vi "Read Trace.vi"(0 "VISA resource name":refnum<visa-resource-name>, 1 "Data Source (0: Data Trace)":u16(ring) items=["Data Trace", "Memory Trace"], 2 "Data Type (0: Formatted)":T1(ring), 5 "Measurement Type (6: Phase Noise)":u16(ring)=6 items=["AM Noise"=1, "Baseband Noise"=2, "Freq/Power"=3, "Spectrum"=4, "Transient"=5, "Phase Noise"=6, "User"=7], 7 "Select Trace (1: 1)":u16(ring)=1 items=["1"=1, "2"=2, "3"=3, "4"=4, "5"=5, "6"=6, "7"=7, "8"=8], 11 "error in (no error)":errorcluster, 12 "Maximum Time (10000 ms)":u32=10000) -> (4 "VISA resource name out":refnum<visa-resource-name>, 6 "Measurements":dbl[](array[numeric]) format="%^#_9g", 15 "error out":errorcluster)   [LabVIEW 2011, in "Agilent E5052X.lvlib"]
doc: "Reads formatted trace data from the instrument. \n\n<b>Note: </b>\n\nIt can read either data from current trace or from trace stored in memory."
uses:
  Agilent E5052X.lvlib
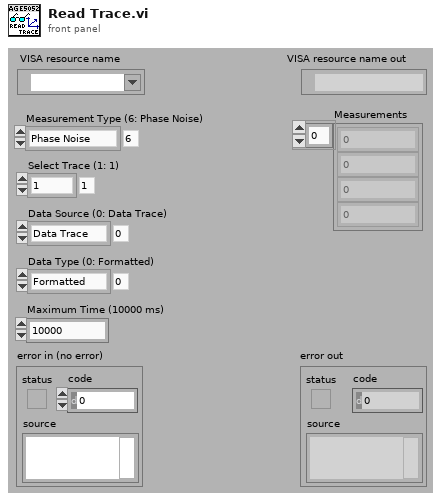
[diagram p1: front panel]
types:
  T1 = enum16{"Formatted", "Unformatted", "Power", "Spurious"}
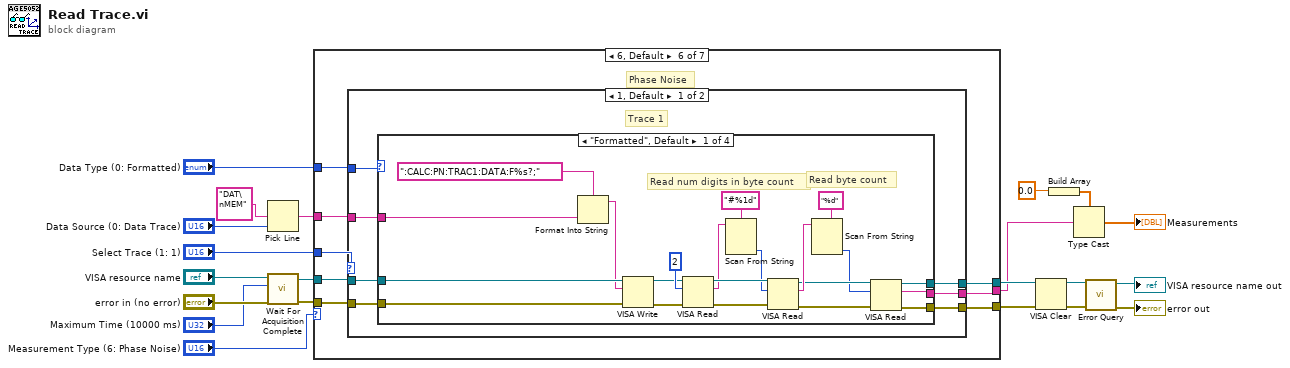
[diagram p0: block diagram]
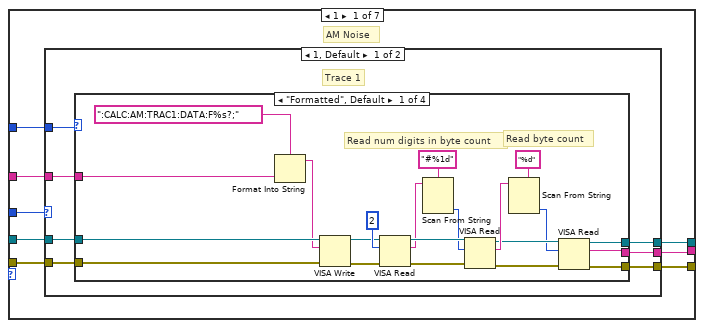
[diagram p2: hidden frame]
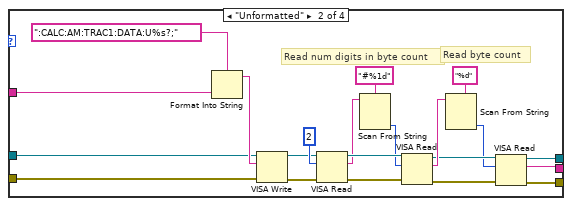
[diagram p3: hidden frame]
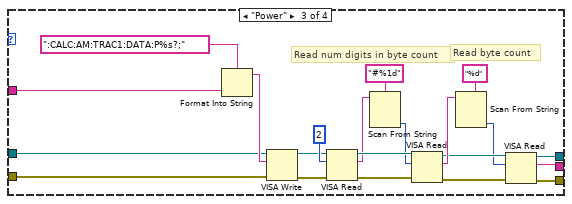
[diagram p4: hidden frame]
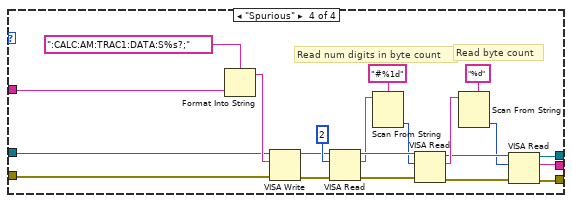
[diagram p5: hidden frame]
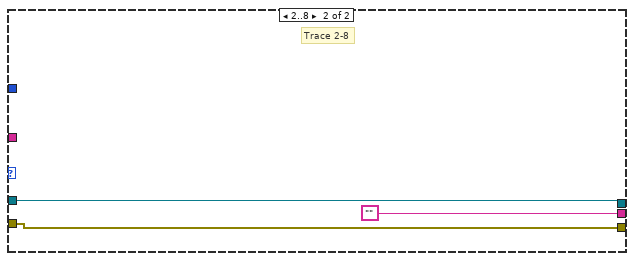
[diagram p6: hidden frame]
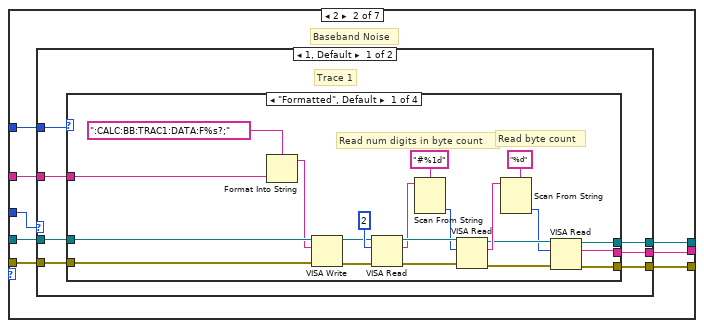
[diagram p7: hidden frame]
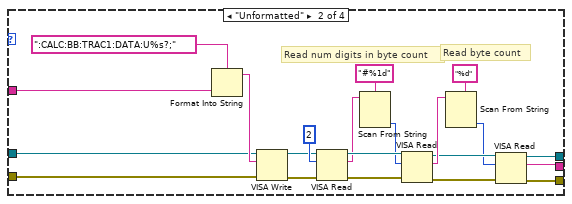
[diagram p8: hidden frame]
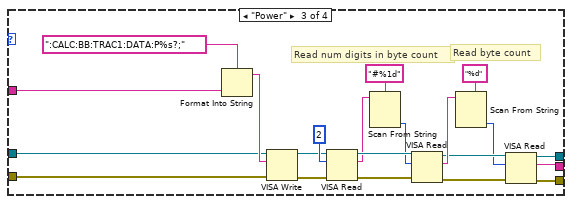
[diagram p9: hidden frame]
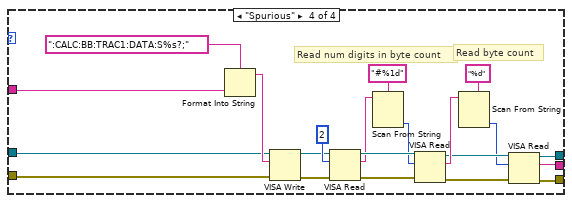
[diagram p10: hidden frame]
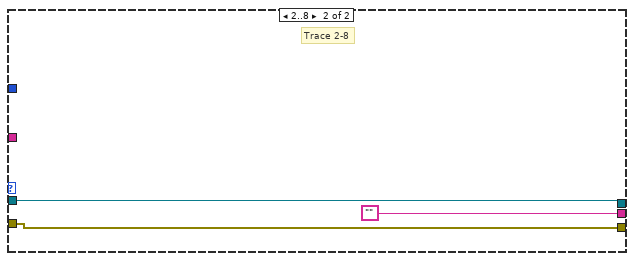
[diagram p11: hidden frame]
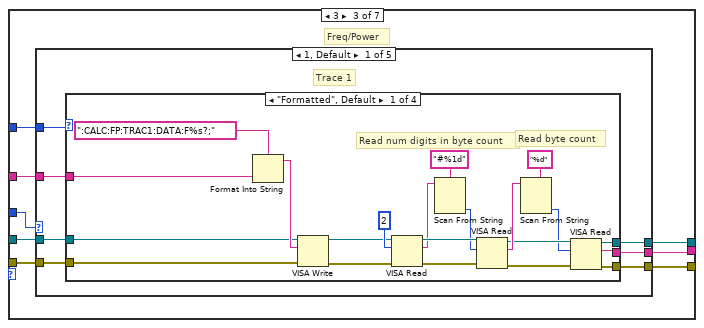
[diagram p12: hidden frame]
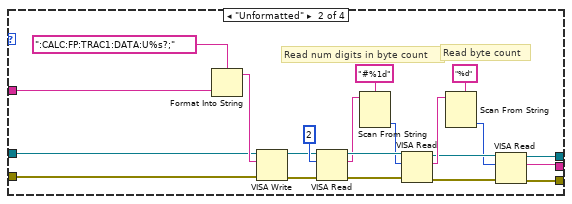
[diagram p13: hidden frame]
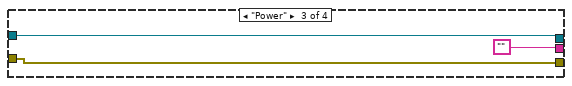
[diagram p14: hidden frame]
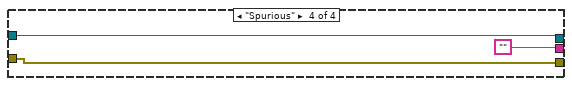
[diagram p15: hidden frame]
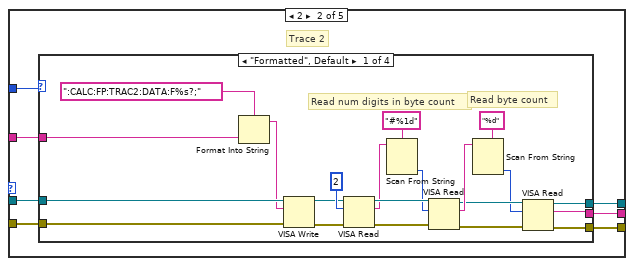
[diagram p16: hidden frame]
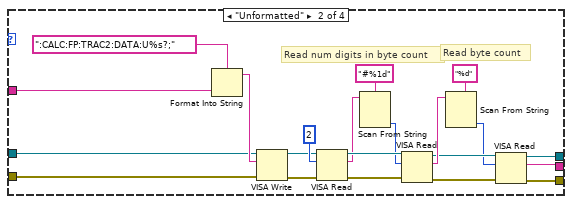
[diagram p17: hidden frame]
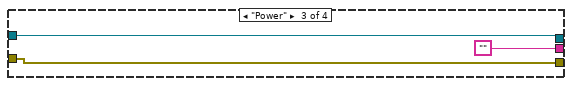
[diagram p18: hidden frame]
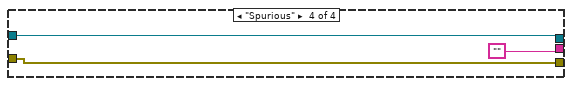
[diagram p19: hidden frame]
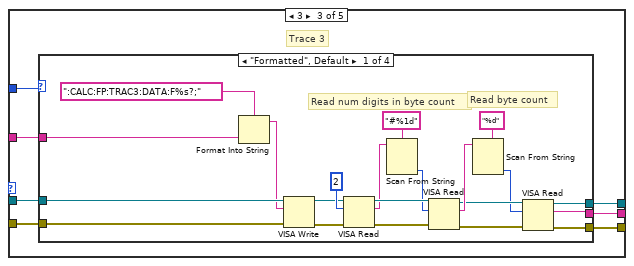
[diagram p20: hidden frame]
diagram:
  n1 = Pick Line(multi-line string="DAT\nMEM", line index="Data Source (0: Data Trace)") -> (output string=w14:string)  [unwired: 1 in]
  n2 = call "Wait For Acquisition Complete.vi"("error in (no error)"="error in (no error)", "Maximum Time (10000)"="Maximum Time (10000 ms)", "VISA resource name"="VISA resource name") -> ("error out"=w8:errorcluster, "VISA resource name out"=w9:refnum<visa-resource-name>)  [unwired: 7 in]
  n3 = case shown="6, Default" "Measurement Type (6: Phase Noise)" {
    tunnel: "Select Trace (1: 1)" -> [w29 w129 w231 w462 w528 w759 w861]
    tunnel: w14 -> [w28 w130 w232 w463 w529 w760 w862]
    tunnel: "Data Type (0: Formatted)" -> [w27 w131 w233 w464 w530 w761 w863]
    tunnel: w9 -> [w26 w128 w230 w461 w527 w758 w860]
    tunnel: w8 -> [w25 w127 w229 w460 w526 w757 w859]
    tunnel: [w24 w126 w228 w459 w525 w756 w858] -> w13
    tunnel: [w23 w124 w226 w457 w523 w754 w856] -> w12
    tunnel: [w22 w125 w227 w458 w524 w755 w857] -> w2
    frame 1 {
      # "AM Noise"
      n4 = case shown="1, Default" w29 {
        tunnel: w28 -> [w35 _]
        tunnel: w27 -> [w36 _]
        tunnel: w26 -> [w34 w122]
        tunnel: w25 -> [w33 w121]
        tunnel: [w32 w122] -> w24
        tunnel: [w31 w121] -> w23
        tunnel: [w30 ""] -> w22
        frame 1, Default {
          # "Trace 1"
          n5 = case shown="\"Formatted\", Default" w36 {
            tunnel: w35 -> [w56 w63 w84 w105]
            tunnel: w34 -> [w55 w62 w83 w104]
            tunnel: w33 -> [w54 w61 w82 w103]
            tunnel: [w52 w60 w81 w102] -> w32
            tunnel: [w51 w59 w79 w101] -> w31
            tunnel: [w50 w58 w80 w100] -> w30
            frame "Formatted", Default {
              # "Read num digits in byte count"
              # "Read byte count"
              n6 = Format Into String(format string=":CALC:AM:TRAC1:DATA:F%s?;", w56) -> (resulting string=w53:string)  [unwired: 2 in, 1 out]
              n7 = VISA Write(VISA resource name=w55, write buffer=w53, error in (no error)=w54) -> (VISA resource name out=w41:refnum<visa-resource-name>, error out=w40:errorcluster)  [unwired: 1 out]
              n8 = VISA Read(VISA resource name=w41, byte count=u32 2, error in (no error)=w40) -> (VISA resource name out=w46:refnum<visa-resource-name>, read buffer=w42:string, error out=w47:errorcluster)  [unwired: 1 out]
              n9 = Scan From String(format string="#%1d", input string=w42) -> (output 1=w45:i32)  [unwired: 3 in, 3 out]
              n10 = VISA Read(VISA resource name=w46, byte count=w45, error in (no error)=w47) -> (VISA resource name out=w39:refnum<visa-resource-name>, read buffer=w44:string, error out=w38:errorcluster)  [unwired: 1 out]
              n11 = Scan From String(format string="%d", input string=w44) -> (output 1=w37:i32)  [unwired: 3 in, 3 out]
              n12 = VISA Read(VISA resource name=w39, byte count=w37, error in (no error)=w38) -> (VISA resource name out=w52:refnum<visa-resource-name>, read buffer=w50:string, error out=w51:errorcluster)  [unwired: 1 out]
            }
            frame "Unformatted" {
              # "Read num digits in byte count"
              # "Read byte count"
              n13 = Format Into String(format string=":CALC:AM:TRAC1:DATA:U%s?;", w63) -> (resulting string=w77:string)  [unwired: 2 in, 1 out]
              n14 = VISA Write(VISA resource name=w62, write buffer=w77, error in (no error)=w61) -> (VISA resource name out=w68:refnum<visa-resource-name>, error out=w67:errorcluster)  [unwired: 1 out]
              n15 = VISA Read(VISA resource name=w68, byte count=u32 2, error in (no error)=w67) -> (VISA resource name out=w73:refnum<visa-resource-name>, read buffer=w69:string, error out=w74:errorcluster)  [unwired: 1 out]
              n16 = Scan From String(format string="#%1d", input string=w69) -> (output 1=w72:i32)  [unwired: 3 in, 3 out]
              n17 = VISA Read(VISA resource name=w73, byte count=w72, error in (no error)=w74) -> (VISA resource name out=w66:refnum<visa-resource-name>, read buffer=w71:string, error out=w65:errorcluster)  [unwired: 1 out]
              n18 = Scan From String(format string="%d", input string=w71) -> (output 1=w64:i32)  [unwired: 3 in, 3 out]
              n19 = VISA Read(VISA resource name=w66, byte count=w64, error in (no error)=w65) -> (VISA resource name out=w60:refnum<visa-resource-name>, read buffer=w58:string, error out=w59:errorcluster)  [unwired: 1 out]
            }
            frame "Power" {
              # "Read num digits in byte count"
              # "Read byte count"
              n20 = Format Into String(format string=":CALC:AM:TRAC1:DATA:P%s?;", w84) -> (resulting string=w98:string)  [unwired: 2 in, 1 out]
              n21 = VISA Write(VISA resource name=w83, write buffer=w98, error in (no error)=w82) -> (VISA resource name out=w89:refnum<visa-resource-name>, error out=w88:errorcluster)  [unwired: 1 out]
              n22 = VISA Read(VISA resource name=w89, byte count=u32 2, error in (no error)=w88) -> (VISA resource name out=w94:refnum<visa-resource-name>, read buffer=w90:string, error out=w95:errorcluster)  [unwired: 1 out]
              n23 = Scan From String(format string="#%1d", input string=w90) -> (output 1=w93:i32)  [unwired: 3 in, 3 out]
              n24 = VISA Read(VISA resource name=w94, byte count=w93, error in (no error)=w95) -> (VISA resource name out=w87:refnum<visa-resource-name>, read buffer=w92:string, error out=w86:errorcluster)  [unwired: 1 out]
              n25 = Scan From String(format string="%d", input string=w92) -> (output 1=w85:i32)  [unwired: 3 in, 3 out]
              n26 = VISA Read(VISA resource name=w87, byte count=w85, error in (no error)=w86) -> (VISA resource name out=w81:refnum<visa-resource-name>, read buffer=w80:string, error out=w79:errorcluster)  [unwired: 1 out]
            }
            frame "Spurious" {
              # "Read num digits in byte count"
              # "Read byte count"
              n27 = Format Into String(format string=":CALC:AM:TRAC1:DATA:S%s?;", w105) -> (resulting string=w119:string)  [unwired: 2 in, 1 out]
              n28 = VISA Write(VISA resource name=w104, write buffer=w119, error in (no error)=w103) -> (VISA resource name out=w110:refnum<visa-resource-name>, error out=w109:errorcluster)  [unwired: 1 out]
              n29 = VISA Read(VISA resource name=w110, byte count=u32 2, error in (no error)=w109) -> (VISA resource name out=w115:refnum<visa-resource-name>, read buffer=w111:string, error out=w116:errorcluster)  [unwired: 1 out]
              n30 = Scan From String(format string="#%1d", input string=w111) -> (output 1=w114:i32)  [unwired: 3 in, 3 out]
              n31 = VISA Read(VISA resource name=w115, byte count=w114, error in (no error)=w116) -> (VISA resource name out=w108:refnum<visa-resource-name>, read buffer=w113:string, error out=w107:errorcluster)  [unwired: 1 out]
              n32 = Scan From String(format string="%d", input string=w113) -> (output 1=w106:i32)  [unwired: 3 in, 3 out]
              n33 = VISA Read(VISA resource name=w108, byte count=w106, error in (no error)=w107) -> (VISA resource name out=w102:refnum<visa-resource-name>, read buffer=w100:string, error out=w101:errorcluster)  [unwired: 1 out]
            }
          }
        }
        frame 2..8 {
          # "Trace 2-8"
        }
      }
    }
    frame 2 {
      # "Baseband Noise"
      n34 = case shown="1, Default" w129 {
        tunnel: w130 -> [w137 _]
        tunnel: w131 -> [w138 _]
        tunnel: w128 -> [w136 w224]
        tunnel: w127 -> [w135 w223]
        tunnel: [w134 w224] -> w126
        tunnel: [w133 w223] -> w124
        tunnel: [w132 ""] -> w125
        frame 1, Default {
          # "Trace 1"
          n35 = case shown="\"Formatted\", Default" w138 {
            tunnel: w137 -> [w158 w165 w186 w207]
            tunnel: w136 -> [w157 w164 w185 w206]
            tunnel: w135 -> [w156 w163 w184 w205]
            tunnel: [w154 w162 w183 w204] -> w134
            tunnel: [w153 w161 w181 w203] -> w133
            tunnel: [w152 w160 w182 w202] -> w132
            frame "Formatted", Default {
              # "Read num digits in byte count"
              # "Read byte count"
              n36 = Format Into String(format string=":CALC:BB:TRAC1:DATA:F%s?;", w158) -> (resulting string=w155:string)  [unwired: 2 in, 1 out]
              n37 = VISA Write(VISA resource name=w157, write buffer=w155, error in (no error)=w156) -> (VISA resource name out=w143:refnum<visa-resource-name>, error out=w142:errorcluster)  [unwired: 1 out]
              n38 = VISA Read(VISA resource name=w143, byte count=u32 2, error in (no error)=w142) -> (VISA resource name out=w148:refnum<visa-resource-name>, read buffer=w144:string, error out=w149:errorcluster)  [unwired: 1 out]
              n39 = Scan From String(format string="#%1d", input string=w144) -> (output 1=w147:i32)  [unwired: 3 in, 3 out]
              n40 = VISA Read(VISA resource name=w148, byte count=w147, error in (no error)=w149) -> (VISA resource name out=w141:refnum<visa-resource-name>, read buffer=w146:string, error out=w140:errorcluster)  [unwired: 1 out]
              n41 = Scan From String(format string="%d", input string=w146) -> (output 1=w139:i32)  [unwired: 3 in, 3 out]
              n42 = VISA Read(VISA resource name=w141, byte count=w139, error in (no error)=w140) -> (VISA resource name out=w154:refnum<visa-resource-name>, read buffer=w152:string, error out=w153:errorcluster)  [unwired: 1 out]
            }
            frame "Unformatted" {
              # "Read num digits in byte count"
              # "Read byte count"
              n43 = Format Into String(format string=":CALC:BB:TRAC1:DATA:U%s?;", w165) -> (resulting string=w179:string)  [unwired: 2 in, 1 out]
              n44 = VISA Write(VISA resource name=w164, write buffer=w179, error in (no error)=w163) -> (VISA resource name out=w170:refnum<visa-resource-name>, error out=w169:errorcluster)  [unwired: 1 out]
              n45 = VISA Read(VISA resource name=w170, byte count=u32 2, error in (no error)=w169) -> (VISA resource name out=w175:refnum<visa-resource-name>, read buffer=w171:string, error out=w176:errorcluster)  [unwired: 1 out]
              n46 = Scan From String(format string="#%1d", input string=w171) -> (output 1=w174:i32)  [unwired: 3 in, 3 out]
              n47 = VISA Read(VISA resource name=w175, byte count=w174, error in (no error)=w176) -> (VISA resource name out=w168:refnum<visa-resource-name>, read buffer=w173:string, error out=w167:errorcluster)  [unwired: 1 out]
              n48 = Scan From String(format string="%d", input string=w173) -> (output 1=w166:i32)  [unwired: 3 in, 3 out]
              n49 = VISA Read(VISA resource name=w168, byte count=w166, error in (no error)=w167) -> (VISA resource name out=w162:refnum<visa-resource-name>, read buffer=w160:string, error out=w161:errorcluster)  [unwired: 1 out]
            }
            frame "Power" {
              # "Read num digits in byte count"
              # "Read byte count"
              n50 = Format Into String(format string=":CALC:BB:TRAC1:DATA:P%s?;", w186) -> (resulting string=w200:string)  [unwired: 2 in, 1 out]
              n51 = VISA Write(VISA resource name=w185, write buffer=w200, error in (no error)=w184) -> (VISA resource name out=w191:refnum<visa-resource-name>, error out=w190:errorcluster)  [unwired: 1 out]
              n52 = VISA Read(VISA resource name=w191, byte count=u32 2, error in (no error)=w190) -> (VISA resource name out=w196:refnum<visa-resource-name>, read buffer=w192:string, error out=w197:errorcluster)  [unwired: 1 out]
              n53 = Scan From String(format string="#%1d", input string=w192) -> (output 1=w195:i32)  [unwired: 3 in, 3 out]
              n54 = VISA Read(VISA resource name=w196, byte count=w195, error in (no error)=w197) -> (VISA resource name out=w189:refnum<visa-resource-name>, read buffer=w194:string, error out=w188:errorcluster)  [unwired: 1 out]
              n55 = Scan From String(format string="%d", input string=w194) -> (output 1=w187:i32)  [unwired: 3 in, 3 out]
              n56 = VISA Read(VISA resource name=w189, byte count=w187, error in (no error)=w188) -> (VISA resource name out=w183:refnum<visa-resource-name>, read buffer=w182:string, error out=w181:errorcluster)  [unwired: 1 out]
            }
            frame "Spurious" {
              # "Read num digits in byte count"
              # "Read byte count"
              n57 = Format Into String(format string=":CALC:BB:TRAC1:DATA:S%s?;", w207) -> (resulting string=w221:string)  [unwired: 2 in, 1 out]
              n58 = VISA Write(VISA resource name=w206, write buffer=w221, error in (no error)=w205) -> (VISA resource name out=w212:refnum<visa-resource-name>, error out=w211:errorcluster)  [unwired: 1 out]
              n59 = VISA Read(VISA resource name=w212, byte count=u32 2, error in (no error)=w211) -> (VISA resource name out=w217:refnum<visa-resource-name>, read buffer=w213:string, error out=w218:errorcluster)  [unwired: 1 out]
              n60 = Scan From String(format string="#%1d", input string=w213) -> (output 1=w216:i32)  [unwired: 3 in, 3 out]
              n61 = VISA Read(VISA resource name=w217, byte count=w216, error in (no error)=w218) -> (VISA resource name out=w210:refnum<visa-resource-name>, read buffer=w215:string, error out=w209:errorcluster)  [unwired: 1 out]
              n62 = Scan From String(format string="%d", input string=w215) -> (output 1=w208:i32)  [unwired: 3 in, 3 out]
              n63 = VISA Read(VISA resource name=w210, byte count=w208, error in (no error)=w209) -> (VISA resource name out=w204:refnum<visa-resource-name>, read buffer=w202:string, error out=w203:errorcluster)  [unwired: 1 out]
            }
          }
        }
        frame 2..8 {
          # "Trace 2-8"
        }
      }
    }
    frame 3 {
      # "Freq/Power"
      n64 = case shown="1, Default" w231 {
        tunnel: w232 -> [w239 w294 w349 w404 _]
        tunnel: w233 -> [w240 w295 w350 w405 _]
        tunnel: w230 -> [w238 w293 w348 w403 w456]
        tunnel: w229 -> [w237 w292 w347 w402 w455]
        tunnel: [w236 w291 w346 w401 w456] -> w228
        tunnel: [w235 w290 w345 w400 w455] -> w226
        tunnel: [w234 w289 w344 w399 ""] -> w227
        frame 1, Default {
          # "Trace 1"
          n65 = case shown="\"Formatted\", Default" w240 {
            tunnel: w239 -> [w260 w267 _ _]
            tunnel: w238 -> [w242 w266 w285 w288]
            tunnel: w237 -> [w241 w265 w284 w287]
            tunnel: [w258 w264 w285 w288] -> w236
            tunnel: [w257 w263 w284 w287] -> w235
            tunnel: [w256 w262 "" ""] -> w234
            frame "Formatted", Default {
              # "Read num digits in byte count"
              # "Read byte count"
              n66 = Format Into String(format string=":CALC:FP:TRAC1:DATA:F%s?;", w260) -> (resulting string=w259:string)  [unwired: 2 in, 1 out]
              n67 = VISA Write(VISA resource name=w242, write buffer=w259, error in (no error)=w241) -> (VISA resource name out=w244:refnum<visa-resource-name>, error out=w243:errorcluster)  [unwired: 1 out]
              n68 = VISA Read(VISA resource name=w244, byte count=u32 2, error in (no error)=w243) -> (VISA resource name out=w252:refnum<visa-resource-name>, read buffer=w248:string, error out=w253:errorcluster)  [unwired: 1 out]
              n69 = Scan From String(format string="#%1d", input string=w248) -> (output 1=w251:i32)  [unwired: 3 in, 3 out]
              n70 = VISA Read(VISA resource name=w252, byte count=w251, error in (no error)=w253) -> (VISA resource name out=w247:refnum<visa-resource-name>, read buffer=w250:string, error out=w246:errorcluster)  [unwired: 1 out]
              n71 = Scan From String(format string="%d", input string=w250) -> (output 1=w245:i32)  [unwired: 3 in, 3 out]
              n72 = VISA Read(VISA resource name=w247, byte count=w245, error in (no error)=w246) -> (VISA resource name out=w258:refnum<visa-resource-name>, read buffer=w256:string, error out=w257:errorcluster)  [unwired: 1 out]
            }
            frame "Unformatted" {
              # "Read num digits in byte count"
              # "Read byte count"
              n73 = Format Into String(format string=":CALC:FP:TRAC1:DATA:U%s?;", w267) -> (resulting string=w281:string)  [unwired: 2 in, 1 out]
              n74 = VISA Write(VISA resource name=w266, write buffer=w281, error in (no error)=w265) -> (VISA resource name out=w272:refnum<visa-resource-name>, error out=w271:errorcluster)  [unwired: 1 out]
              n75 = VISA Read(VISA resource name=w272, byte count=u32 2, error in (no error)=w271) -> (VISA resource name out=w277:refnum<visa-resource-name>, read buffer=w273:string, error out=w278:errorcluster)  [unwired: 1 out]
              n76 = Scan From String(format string="#%1d", input string=w273) -> (output 1=w276:i32)  [unwired: 3 in, 3 out]
              n77 = VISA Read(VISA resource name=w277, byte count=w276, error in (no error)=w278) -> (VISA resource name out=w270:refnum<visa-resource-name>, read buffer=w275:string, error out=w269:errorcluster)  [unwired: 1 out]
              n78 = Scan From String(format string="%d", input string=w275) -> (output 1=w268:i32)  [unwired: 3 in, 3 out]
              n79 = VISA Read(VISA resource name=w270, byte count=w268, error in (no error)=w269) -> (VISA resource name out=w264:refnum<visa-resource-name>, read buffer=w262:string, error out=w263:errorcluster)  [unwired: 1 out]
            }
            frame "Power" {
            }
            frame "Spurious" {
            }
          }
        }
        frame 2 {
          # "Trace 2"
          n80 = case shown="\"Formatted\", Default" w295 {
            tunnel: w294 -> [w315 w322 _ _]
            tunnel: w293 -> [w314 w321 w340 w343]
            tunnel: w292 -> [w313 w320 w339 w342]
            tunnel: [w311 w319 w340 w343] -> w291
            tunnel: [w310 w318 w339 w342] -> w290
            tunnel: [w309 w317 "" ""] -> w289
            frame "Formatted", Default {
              # "Read num digits in byte count"
              # "Read byte count"
              n81 = Format Into String(format string=":CALC:FP:TRAC2:DATA:F%s?;", w315) -> (resulting string=w312:string)  [unwired: 2 in, 1 out]
              n82 = VISA Write(VISA resource name=w314, write buffer=w312, error in (no error)=w313) -> (VISA resource name out=w300:refnum<visa-resource-name>, error out=w299:errorcluster)  [unwired: 1 out]
              n83 = VISA Read(VISA resource name=w300, byte count=u32 2, error in (no error)=w299) -> (VISA resource name out=w305:refnum<visa-resource-name>, read buffer=w301:string, error out=w306:errorcluster)  [unwired: 1 out]
              n84 = Scan From String(format string="#%1d", input string=w301) -> (output 1=w304:i32)  [unwired: 3 in, 3 out]
              n85 = VISA Read(VISA resource name=w305, byte count=w304, error in (no error)=w306) -> (VISA resource name out=w298:refnum<visa-resource-name>, read buffer=w303:string, error out=w297:errorcluster)  [unwired: 1 out]
              n86 = Scan From String(format string="%d", input string=w303) -> (output 1=w296:i32)  [unwired: 3 in, 3 out]
              n87 = VISA Read(VISA resource name=w298, byte count=w296, error in (no error)=w297) -> (VISA resource name out=w311:refnum<visa-resource-name>, read buffer=w309:string, error out=w310:errorcluster)  [unwired: 1 out]
            }
            frame "Unformatted" {
              # "Read num digits in byte count"
              # "Read byte count"
              n88 = Format Into String(format string=":CALC:FP:TRAC2:DATA:U%s?;", w322) -> (resulting string=w336:string)  [unwired: 2 in, 1 out]
              n89 = VISA Write(VISA resource name=w321, write buffer=w336, error in (no error)=w320) -> (VISA resource name out=w327:refnum<visa-resource-name>, error out=w326:errorcluster)  [unwired: 1 out]
              n90 = VISA Read(VISA resource name=w327, byte count=u32 2, error in (no error)=w326) -> (VISA resource name out=w332:refnum<visa-resource-name>, read buffer=w328:string, error out=w333:errorcluster)  [unwired: 1 out]
              n91 = Scan From String(format string="#%1d", input string=w328) -> (output 1=w331:i32)  [unwired: 3 in, 3 out]
              n92 = VISA Read(VISA resource name=w332, byte count=w331, error in (no error)=w333) -> (VISA resource name out=w325:refnum<visa-resource-name>, read buffer=w330:string, error out=w324:errorcluster)  [unwired: 1 out]
              n93 = Scan From String(format string="%d", input string=w330) -> (output 1=w323:i32)  [unwired: 3 in, 3 out]
              n94 = VISA Read(VISA resource name=w325, byte count=w323, error in (no error)=w324) -> (VISA resource name out=w319:refnum<visa-resource-name>, read buffer=w317:string, error out=w318:errorcluster)  [unwired: 1 out]
            }
            frame "Power" {
            }
            frame "Spurious" {
            }
          }
        }
        frame 3 {
          # "Trace 3"
          n95 = case shown="\"Formatted\", Default" w350 {
            tunnel: w349 -> [w370 w377 _ _]
            tunnel: w348 -> [w369 w376 w395 w398]
            tunnel: w347 -> [w368 w375 w394 w397]
            tunnel: [w366 w374 w395 w398] -> w346
            tunnel: [w365 w373 w394 w397] -> w345
            tunnel: [w364 w372 "" ""] -> w344
            frame "Formatted", Default {
              # "Read num digits in byte count"
              # "Read byte count"
              n96 = Format Into String(format string=":CALC:FP:TRAC3:DATA:F%s?;", w370) -> (resulting string=w367:string)  [unwired: 2 in, 1 out]
              n97 = VISA Write(VISA resource name=w369, write buffer=w367, error in (no error)=w368) -> (VISA resource name out=w355:refnum<visa-resource-name>, error out=w354:errorcluster)  [unwired: 1 out]
              n98 = VISA Read(VISA resource name=w355, byte count=u32 2, error in (no error)=w354) -> (VISA resource name out=w360:refnum<visa-resource-name>, read buffer=w356:string, error out=w361:errorcluster)  [unwired: 1 out]
              n99 = Scan From String(format string="#%1d", input string=w356) -> (output 1=w359:i32)  [unwired: 3 in, 3 out]
              n100 = VISA Read(VISA resource name=w360, byte count=w359, error in (no error)=w361) -> (VISA resource name out=w353:refnum<visa-resource-name>, read buffer=w358:string, error out=w352:errorcluster)  [unwired: 1 out]
              n101 = Scan From String(format string="%d", input string=w358) -> (output 1=w351:i32)  [unwired: 3 in, 3 out]
              n102 = VISA Read(VISA resource name=w353, byte count=w351, error in (no error)=w352) -> (VISA resource name out=w366:refnum<visa-resource-name>, read buffer=w364:string, error out=w365:errorcluster)  [unwired: 1 out]
            }
            frame "Unformatted" {
              # "Read num digits in byte count"
              # "Read byte count"
              n103 = Format Into String(format string=":CALC:FP:TRAC3:DATA:U%s?;", w377) -> (resulting string=w391:string)  [unwired: 2 in, 1 out]
              n104 = VISA Write(VISA resource name=w376, write buffer=w391, error in (no error)=w375) -> (VISA resource name out=w382:refnum<visa-resource-name>, error out=w381:errorcluster)  [unwired: 1 out]
              n105 = VISA Read(VISA resource name=w382, byte count=u32 2, error in (no error)=w381) -> (VISA resource name out=w387:refnum<visa-resource-name>, read buffer=w383:string, error out=w388:errorcluster)  [unwired: 1 out]
              n106 = Scan From String(format string="#%1d", input string=w383) -> (output 1=w386:i32)  [unwired: 3 in, 3 out]
              n107 = VISA Read(VISA resource name=w387, byte count=w386, error in (no error)=w388) -> (VISA resource name out=w380:refnum<visa-resource-name>, read buffer=w385:string, error out=w379:errorcluster)  [unwired: 1 out]
              n108 = Scan From String(format string="%d", input string=w385) -> (output 1=w378:i32)  [unwired: 3 in, 3 out]
              n109 = VISA Read(VISA resource name=w380, byte count=w378, error in (no error)=w379) -> (VISA resource name out=w374:refnum<visa-resource-name>, read buffer=w372:string, error out=w373:errorcluster)  [unwired: 1 out]
            }
            frame "Power" {
            }
            frame "Spurious" {
            }
          }
        }
        frame 4 {
          # "Trace 4"
          n110 = case shown="\"Formatted\", Default" w405 {
            tunnel: w404 -> [w425 w432 _ _]
            tunnel: w403 -> [w424 w431 w450 w453]
            tunnel: w402 -> [w423 w430 w449 w452]
            tunnel: [w421 w429 w450 w453] -> w401
            tunnel: [w420 w428 w449 w452] -> w400
            tunnel: [w419 w427 "" ""] -> w399
            frame "Formatted", Default {
              # "Read num digits in byte count"
              # "Read byte count"
              n111 = Format Into String(format string=":CALC:FP:TRAC4:DATA:F%s?;", w425) -> (resulting string=w422:string)  [unwired: 2 in, 1 out]
              n112 = VISA Write(VISA resource name=w424, write buffer=w422, error in (no error)=w423) -> (VISA resource name out=w410:refnum<visa-resource-name>, error out=w409:errorcluster)  [unwired: 1 out]
              n113 = VISA Read(VISA resource name=w410, byte count=u32 2, error in (no error)=w409) -> (VISA resource name out=w415:refnum<visa-resource-name>, read buffer=w411:string, error out=w416:errorcluster)  [unwired: 1 out]
              n114 = Scan From String(format string="#%1d", input string=w411) -> (output 1=w414:i32)  [unwired: 3 in, 3 out]
              n115 = VISA Read(VISA resource name=w415, byte count=w414, error in (no error)=w416) -> (VISA resource name out=w408:refnum<visa-resource-name>, read buffer=w413:string, error out=w407:errorcluster)  [unwired: 1 out]
              n116 = Scan From String(format string="%d", input string=w413) -> (output 1=w406:i32)  [unwired: 3 in, 3 out]
              n117 = VISA Read(VISA resource name=w408, byte count=w406, error in (no error)=w407) -> (VISA resource name out=w421:refnum<visa-resource-name>, read buffer=w419:string, error out=w420:errorcluster)  [unwired: 1 out]
            }
            frame "Unformatted" {
              # "Read num digits in byte count"
              # "Read byte count"
              n118 = Format Into String(format string=":CALC:FP:TRAC4:DATA:U%s?;", w432) -> (resulting string=w446:string)  [unwired: 2 in, 1 out]
              n119 = VISA Write(VISA resource name=w431, write buffer=w446, error in (no error)=w430) -> (VISA resource name out=w437:refnum<visa-resource-name>, error out=w436:errorcluster)  [unwired: 1 out]
              n120 = VISA Read(VISA resource name=w437, byte count=u32 2, error in (no error)=w436) -> (VISA resource name out=w442:refnum<visa-resource-name>, read buffer=w438:string, error out=w443:errorcluster)  [unwired: 1 out]
              n121 = Scan From String(format string="#%1d", input string=w438) -> (output 1=w441:i32)  [unwired: 3 in, 3 out]
              n122 = VISA Read(VISA resource name=w442, byte count=w441, error in (no error)=w443) -> (VISA resource name out=w435:refnum<visa-resource-name>, read buffer=w440:string, error out=w434:errorcluster)  [unwired: 1 out]
              n123 = Scan From String(format string="%d", input string=w440) -> (output 1=w433:i32)  [unwired: 3 in, 3 out]
              n124 = VISA Read(VISA resource name=w435, byte count=w433, error in (no error)=w434) -> (VISA resource name out=w429:refnum<visa-resource-name>, read buffer=w427:string, error out=w428:errorcluster)  [unwired: 1 out]
            }
            frame "Power" {
            }
            frame "Spurious" {
            }
          }
        }
        frame 5..8 {
        }
      }
    }
    frame 4 {
      # "Spectrum"
      n125 = case shown="1, Default" w462 {
        tunnel: w463 -> [w470 _]
        tunnel: w464 -> [w471 _]
        tunnel: w461 -> [w469 w521]
        tunnel: w460 -> [w468 w520]
        tunnel: [w467 w521] -> w459
        tunnel: [w466 w520] -> w457
        tunnel: [w465 ""] -> w458
        frame 1, Default {
          # "Trace 1"
          n126 = case shown="\"Formatted\", Default" w471 {
            tunnel: w470 -> [w491 w498 _ _]
            tunnel: w469 -> [w490 w497 w516 w519]
            tunnel: w468 -> [w489 w496 w515 w518]
            tunnel: [w487 w495 w516 w519] -> w467
            tunnel: [w486 w494 w515 w518] -> w466
            tunnel: [w485 w493 "" ""] -> w465
            frame "Formatted", Default {
              # "Read num digits in byte count"
              # "Read byte count"
              n127 = Format Into String(format string=":CALC:SP:TRAC1:DATA:F%s?;", w491) -> (resulting string=w488:string)  [unwired: 2 in, 1 out]
              n128 = VISA Write(VISA resource name=w490, write buffer=w488, error in (no error)=w489) -> (VISA resource name out=w476:refnum<visa-resource-name>, error out=w475:errorcluster)  [unwired: 1 out]
              n129 = VISA Read(VISA resource name=w476, byte count=u32 2, error in (no error)=w475) -> (VISA resource name out=w481:refnum<visa-resource-name>, read buffer=w477:string, error out=w482:errorcluster)  [unwired: 1 out]
              n130 = Scan From String(format string="#%1d", input string=w477) -> (output 1=w480:i32)  [unwired: 3 in, 3 out]
              n131 = VISA Read(VISA resource name=w481, byte count=w480, error in (no error)=w482) -> (VISA resource name out=w474:refnum<visa-resource-name>, read buffer=w479:string, error out=w473:errorcluster)  [unwired: 1 out]
              n132 = Scan From String(format string="%d", input string=w479) -> (output 1=w472:i32)  [unwired: 3 in, 3 out]
              n133 = VISA Read(VISA resource name=w474, byte count=w472, error in (no error)=w473) -> (VISA resource name out=w487:refnum<visa-resource-name>, read buffer=w485:string, error out=w486:errorcluster)  [unwired: 1 out]
            }
            frame "Unformatted" {
              # "Read num digits in byte count"
              # "Read byte count"
              n134 = Format Into String(format string=":CALC:SP:TRAC1:DATA:U%s?;", w498) -> (resulting string=w512:string)  [unwired: 2 in, 1 out]
              n135 = VISA Write(VISA resource name=w497, write buffer=w512, error in (no error)=w496) -> (VISA resource name out=w503:refnum<visa-resource-name>, error out=w502:errorcluster)  [unwired: 1 out]
              n136 = VISA Read(VISA resource name=w503, byte count=u32 2, error in (no error)=w502) -> (VISA resource name out=w508:refnum<visa-resource-name>, read buffer=w504:string, error out=w509:errorcluster)  [unwired: 1 out]
              n137 = Scan From String(format string="#%1d", input string=w504) -> (output 1=w507:i32)  [unwired: 3 in, 3 out]
              n138 = VISA Read(VISA resource name=w508, byte count=w507, error in (no error)=w509) -> (VISA resource name out=w501:refnum<visa-resource-name>, read buffer=w506:string, error out=w500:errorcluster)  [unwired: 1 out]
              n139 = Scan From String(format string="%d", input string=w506) -> (output 1=w499:i32)  [unwired: 3 in, 3 out]
              n140 = VISA Read(VISA resource name=w501, byte count=w499, error in (no error)=w500) -> (VISA resource name out=w495:refnum<visa-resource-name>, read buffer=w493:string, error out=w494:errorcluster)  [unwired: 1 out]
            }
            frame "Power" {
            }
            frame "Spurious" {
            }
          }
        }
        frame 2..8 {
          # "Trace 2-8"
        }
      }
    }
    frame 5 {
      # "Transient"
      n141 = case shown="1, Default" w528 {
        tunnel: w529 -> [w536 w591 w646 w701 _]
        tunnel: w530 -> [w537 w592 w647 w702 _]
        tunnel: w527 -> [w535 w590 w645 w700 w753]
        tunnel: w526 -> [w534 w589 w644 w699 w752]
        tunnel: [w533 w588 w643 w698 w753] -> w525
        tunnel: [w532 w587 w642 w697 w752] -> w523
        tunnel: [w531 w586 w641 w696 ""] -> w524
        frame 1, Default {
          # "Trace 1"
          n142 = case shown="\"Formatted\", Default" w537 {
            tunnel: w536 -> [w557 w564 _ _]
            tunnel: w535 -> [w556 w563 w582 w585]
            tunnel: w534 -> [w555 w562 w581 w584]
            tunnel: [w553 w561 w582 w585] -> w533
            tunnel: [w552 w560 w581 w584] -> w532
            tunnel: [w551 w559 "" ""] -> w531
            frame "Formatted", Default {
              # "Read num digits in byte count"
              # "Read byte count"
              n143 = Format Into String(format string=":CALC:TR:TRAC1:DATA:F%s?;", w557) -> (resulting string=w554:string)  [unwired: 2 in, 1 out]
              n144 = VISA Write(VISA resource name=w556, write buffer=w554, error in (no error)=w555) -> (VISA resource name out=w542:refnum<visa-resource-name>, error out=w541:errorcluster)  [unwired: 1 out]
              n145 = VISA Read(VISA resource name=w542, byte count=u32 2, error in (no error)=w541) -> (VISA resource name out=w547:refnum<visa-resource-name>, read buffer=w543:string, error out=w548:errorcluster)  [unwired: 1 out]
              n146 = Scan From String(format string="#%1d", input string=w543) -> (output 1=w546:i32)  [unwired: 3 in, 3 out]
              n147 = VISA Read(VISA resource name=w547, byte count=w546, error in (no error)=w548) -> (VISA resource name out=w540:refnum<visa-resource-name>, read buffer=w545:string, error out=w539:errorcluster)  [unwired: 1 out]
              n148 = Scan From String(format string="%d", input string=w545) -> (output 1=w538:i32)  [unwired: 3 in, 3 out]
              n149 = VISA Read(VISA resource name=w540, byte count=w538, error in (no error)=w539) -> (VISA resource name out=w553:refnum<visa-resource-name>, read buffer=w551:string, error out=w552:errorcluster)  [unwired: 1 out]
            }
            frame "Unformatted" {
              # "Read num digits in byte count"
              # "Read byte count"
              n150 = Format Into String(format string=":CALC:TR:TRAC1:DATA:U%s?;", w564) -> (resulting string=w578:string)  [unwired: 2 in, 1 out]
              n151 = VISA Write(VISA resource name=w563, write buffer=w578, error in (no error)=w562) -> (VISA resource name out=w569:refnum<visa-resource-name>, error out=w568:errorcluster)  [unwired: 1 out]
              n152 = VISA Read(VISA resource name=w569, byte count=u32 2, error in (no error)=w568) -> (VISA resource name out=w574:refnum<visa-resource-name>, read buffer=w570:string, error out=w575:errorcluster)  [unwired: 1 out]
              n153 = Scan From String(format string="#%1d", input string=w570) -> (output 1=w573:i32)  [unwired: 3 in, 3 out]
              n154 = VISA Read(VISA resource name=w574, byte count=w573, error in (no error)=w575) -> (VISA resource name out=w567:refnum<visa-resource-name>, read buffer=w572:string, error out=w566:errorcluster)  [unwired: 1 out]
              n155 = Scan From String(format string="%d", input string=w572) -> (output 1=w565:i32)  [unwired: 3 in, 3 out]
              n156 = VISA Read(VISA resource name=w567, byte count=w565, error in (no error)=w566) -> (VISA resource name out=w561:refnum<visa-resource-name>, read buffer=w559:string, error out=w560:errorcluster)  [unwired: 1 out]
            }
            frame "Power" {
            }
            frame "Spurious" {
            }
          }
        }
        frame 2 {
          # "Trace 2"
          n157 = case shown="\"Formatted\", Default" w592 {
            tunnel: w591 -> [w612 w619 _ _]
            tunnel: w590 -> [w611 w618 w637 w640]
            tunnel: w589 -> [w610 w617 w636 w639]
            tunnel: [w608 w616 w637 w640] -> w588
            tunnel: [w607 w615 w636 w639] -> w587
            tunnel: [w606 w614 "" ""] -> w586
            frame "Formatted", Default {
              # "Read num digits in byte count"
              # "Read byte count"
              n158 = Format Into String(format string=":CALC:TR:TRAC2:DATA:F%s?;", w612) -> (resulting string=w609:string)  [unwired: 2 in, 1 out]
              n159 = VISA Write(VISA resource name=w611, write buffer=w609, error in (no error)=w610) -> (VISA resource name out=w597:refnum<visa-resource-name>, error out=w596:errorcluster)  [unwired: 1 out]
              n160 = VISA Read(VISA resource name=w597, byte count=u32 2, error in (no error)=w596) -> (VISA resource name out=w602:refnum<visa-resource-name>, read buffer=w598:string, error out=w603:errorcluster)  [unwired: 1 out]
              n161 = Scan From String(format string="#%1d", input string=w598) -> (output 1=w601:i32)  [unwired: 3 in, 3 out]
              n162 = VISA Read(VISA resource name=w602, byte count=w601, error in (no error)=w603) -> (VISA resource name out=w595:refnum<visa-resource-name>, read buffer=w600:string, error out=w594:errorcluster)  [unwired: 1 out]
              n163 = Scan From String(format string="%d", input string=w600) -> (output 1=w593:i32)  [unwired: 3 in, 3 out]
              n164 = VISA Read(VISA resource name=w595, byte count=w593, error in (no error)=w594) -> (VISA resource name out=w608:refnum<visa-resource-name>, read buffer=w606:string, error out=w607:errorcluster)  [unwired: 1 out]
            }
            frame "Unformatted" {
              # "Read num digits in byte count"
              # "Read byte count"
              n165 = Format Into String(format string=":CALC:TR:TRAC2:DATA:U%s?;", w619) -> (resulting string=w633:string)  [unwired: 2 in, 1 out]
              n166 = VISA Write(VISA resource name=w618, write buffer=w633, error in (no error)=w617) -> (VISA resource name out=w624:refnum<visa-resource-name>, error out=w623:errorcluster)  [unwired: 1 out]
              n167 = VISA Read(VISA resource name=w624, byte count=u32 2, error in (no error)=w623) -> (VISA resource name out=w629:refnum<visa-resource-name>, read buffer=w625:string, error out=w630:errorcluster)  [unwired: 1 out]
              n168 = Scan From String(format string="#%1d", input string=w625) -> (output 1=w628:i32)  [unwired: 3 in, 3 out]
              n169 = VISA Read(VISA resource name=w629, byte count=w628, error in (no error)=w630) -> (VISA resource name out=w622:refnum<visa-resource-name>, read buffer=w627:string, error out=w621:errorcluster)  [unwired: 1 out]
              n170 = Scan From String(format string="%d", input string=w627) -> (output 1=w620:i32)  [unwired: 3 in, 3 out]
              n171 = VISA Read(VISA resource name=w622, byte count=w620, error in (no error)=w621) -> (VISA resource name out=w616:refnum<visa-resource-name>, read buffer=w614:string, error out=w615:errorcluster)  [unwired: 1 out]
            }
            frame "Power" {
            }
            frame "Spurious" {
            }
          }
        }
        frame 3 {
          # "Trace 3"
          n172 = case shown="\"Formatted\", Default" w647 {
            tunnel: w646 -> [w667 w674 _ _]
            tunnel: w645 -> [w666 w673 w692 w695]
            tunnel: w644 -> [w665 w672 w691 w694]
            tunnel: [w663 w671 w692 w695] -> w643
            tunnel: [w662 w670 w691 w694] -> w642
            tunnel: [w661 w669 "" ""] -> w641
            frame "Formatted", Default {
              # "Read num digits in byte count"
              # "Read byte count"
              n173 = Format Into String(format string=":CALC:TR:TRAC3:DATA:F%s?;", w667) -> (resulting string=w664:string)  [unwired: 2 in, 1 out]
              n174 = VISA Write(VISA resource name=w666, write buffer=w664, error in (no error)=w665) -> (VISA resource name out=w652:refnum<visa-resource-name>, error out=w651:errorcluster)  [unwired: 1 out]
              n175 = VISA Read(VISA resource name=w652, byte count=u32 2, error in (no error)=w651) -> (VISA resource name out=w657:refnum<visa-resource-name>, read buffer=w653:string, error out=w658:errorcluster)  [unwired: 1 out]
              n176 = Scan From String(format string="#%1d", input string=w653) -> (output 1=w656:i32)  [unwired: 3 in, 3 out]
              n177 = VISA Read(VISA resource name=w657, byte count=w656, error in (no error)=w658) -> (VISA resource name out=w650:refnum<visa-resource-name>, read buffer=w655:string, error out=w649:errorcluster)  [unwired: 1 out]
              n178 = Scan From String(format string="%d", input string=w655) -> (output 1=w648:i32)  [unwired: 3 in, 3 out]
              n179 = VISA Read(VISA resource name=w650, byte count=w648, error in (no error)=w649) -> (VISA resource name out=w663:refnum<visa-resource-name>, read buffer=w661:string, error out=w662:errorcluster)  [unwired: 1 out]
            }
            frame "Unformatted" {
              # "Read num digits in byte count"
              # "Read byte count"
              n180 = Format Into String(format string=":CALC:TR:TRAC3:DATA:U%s?;", w674) -> (resulting string=w688:string)  [unwired: 2 in, 1 out]
              n181 = VISA Write(VISA resource name=w673, write buffer=w688, error in (no error)=w672) -> (VISA resource name out=w679:refnum<visa-resource-name>, error out=w678:errorcluster)  [unwired: 1 out]
              n182 = VISA Read(VISA resource name=w679, byte count=u32 2, error in (no error)=w678) -> (VISA resource name out=w684:refnum<visa-resource-name>, read buffer=w680:string, error out=w685:errorcluster)  [unwired: 1 out]
              n183 = Scan From String(format string="#%1d", input string=w680) -> (output 1=w683:i32)  [unwired: 3 in, 3 out]
              n184 = VISA Read(VISA resource name=w684, byte count=w683, error in (no error)=w685) -> (VISA resource name out=w677:refnum<visa-resource-name>, read buffer=w682:string, error out=w676:errorcluster)  [unwired: 1 out]
              n185 = Scan From String(format string="%d", input string=w682) -> (output 1=w675:i32)  [unwired: 3 in, 3 out]
              n186 = VISA Read(VISA resource name=w677, byte count=w675, error in (no error)=w676) -> (VISA resource name out=w671:refnum<visa-resource-name>, read buffer=w669:string, error out=w670:errorcluster)  [unwired: 1 out]
            }
            frame "Power" {
            }
            frame "Spurious" {
            }
          }
        }
        frame 4 {
          # "Trace 4"
          n187 = case shown="\"Formatted\", Default" w702 {
            tunnel: w701 -> [w722 w729 _ _]
            tunnel: w700 -> [w721 w728 w747 w750]
            tunnel: w699 -> [w720 w727 w746 w749]
            tunnel: [w718 w726 w747 w750] -> w698
            tunnel: [w717 w725 w746 w749] -> w697
            tunnel: [w716 w724 "" ""] -> w696
            frame "Formatted", Default {
              # "Read num digits in byte count"
              # "Read byte count"
              n188 = Format Into String(format string=":CALC:TR:TRAC4:DATA:F%s?;", w722) -> (resulting string=w719:string)  [unwired: 2 in, 1 out]
              n189 = VISA Write(VISA resource name=w721, write buffer=w719, error in (no error)=w720) -> (VISA resource name out=w707:refnum<visa-resource-name>, error out=w706:errorcluster)  [unwired: 1 out]
              n190 = VISA Read(VISA resource name=w707, byte count=u32 2, error in (no error)=w706) -> (VISA resource name out=w712:refnum<visa-resource-name>, read buffer=w708:string, error out=w713:errorcluster)  [unwired: 1 out]
              n191 = Scan From String(format string="#%1d", input string=w708) -> (output 1=w711:i32)  [unwired: 3 in, 3 out]
              n192 = VISA Read(VISA resource name=w712, byte count=w711, error in (no error)=w713) -> (VISA resource name out=w705:refnum<visa-resource-name>, read buffer=w710:string, error out=w704:errorcluster)  [unwired: 1 out]
              n193 = Scan From String(format string="%d", input string=w710) -> (output 1=w703:i32)  [unwired: 3 in, 3 out]
              n194 = VISA Read(VISA resource name=w705, byte count=w703, error in (no error)=w704) -> (VISA resource name out=w718:refnum<visa-resource-name>, read buffer=w716:string, error out=w717:errorcluster)  [unwired: 1 out]
            }
            frame "Unformatted" {
              # "Read num digits in byte count"
              # "Read byte count"
              n195 = Format Into String(format string=":CALC:TR:TRAC4:DATA:U%s?;", w729) -> (resulting string=w743:string)  [unwired: 2 in, 1 out]
              n196 = VISA Write(VISA resource name=w728, write buffer=w743, error in (no error)=w727) -> (VISA resource name out=w734:refnum<visa-resource-name>, error out=w733:errorcluster)  [unwired: 1 out]
              n197 = VISA Read(VISA resource name=w734, byte count=u32 2, error in (no error)=w733) -> (VISA resource name out=w739:refnum<visa-resource-name>, read buffer=w735:string, error out=w740:errorcluster)  [unwired: 1 out]
              n198 = Scan From String(format string="#%1d", input string=w735) -> (output 1=w738:i32)  [unwired: 3 in, 3 out]
              n199 = VISA Read(VISA resource name=w739, byte count=w738, error in (no error)=w740) -> (VISA resource name out=w732:refnum<visa-resource-name>, read buffer=w737:string, error out=w731:errorcluster)  [unwired: 1 out]
              n200 = Scan From String(format string="%d", input string=w737) -> (output 1=w730:i32)  [unwired: 3 in, 3 out]
              n201 = VISA Read(VISA resource name=w732, byte count=w730, error in (no error)=w731) -> (VISA resource name out=w726:refnum<visa-resource-name>, read buffer=w724:string, error out=w725:errorcluster)  [unwired: 1 out]
            }
            frame "Power" {
            }
            frame "Spurious" {
            }
          }
        }
        frame 5..8 {
        }
      }
    }
    frame 6, Default {
      # "Phase Noise"
      n202 = case shown="1, Default" w759 {
        tunnel: w760 -> [w767 _]
        tunnel: w761 -> [w768 _]
        tunnel: w758 -> [w766 w854]
        tunnel: w757 -> [w765 w853]
        tunnel: [w764 w854] -> w756
        tunnel: [w763 w853] -> w754
        tunnel: [w762 ""] -> w755
        frame 1, Default {
          # "Trace 1"
          n203 = case shown="\"Formatted\", Default" w768 {
            tunnel: w767 -> [w788 w795 w816 w837]
            tunnel: w766 -> [w787 w794 w815 w836]
            tunnel: w765 -> [w786 w793 w814 w835]
            tunnel: [w784 w792 w813 w834] -> w764
            tunnel: [w783 w791 w811 w833] -> w763
            tunnel: [w782 w790 w812 w832] -> w762
            frame "Formatted", Default {
              # "Read num digits in byte count"
              # "Read byte count"
              n204 = Format Into String(format string=":CALC:PN:TRAC1:DATA:F%s?;", w788) -> (resulting string=w785:string)  [unwired: 2 in, 1 out]
              n205 = VISA Write(VISA resource name=w787, write buffer=w785, error in (no error)=w786) -> (VISA resource name out=w773:refnum<visa-resource-name>, error out=w772:errorcluster)  [unwired: 1 out]
              n206 = VISA Read(VISA resource name=w773, byte count=u32 2, error in (no error)=w772) -> (VISA resource name out=w778:refnum<visa-resource-name>, read buffer=w774:string, error out=w779:errorcluster)  [unwired: 1 out]
              n207 = Scan From String(format string="#%1d", input string=w774) -> (output 1=w777:i32)  [unwired: 3 in, 3 out]
              n208 = VISA Read(VISA resource name=w778, byte count=w777, error in (no error)=w779) -> (VISA resource name out=w771:refnum<visa-resource-name>, read buffer=w776:string, error out=w770:errorcluster)  [unwired: 1 out]
              n209 = Scan From String(format string="%d", input string=w776) -> (output 1=w769:i32)  [unwired: 3 in, 3 out]
              n210 = VISA Read(VISA resource name=w771, byte count=w769, error in (no error)=w770) -> (VISA resource name out=w784:refnum<visa-resource-name>, read buffer=w782:string, error out=w783:errorcluster)  [unwired: 1 out]
            }
            frame "Unformatted" {
              # "Read num digits in byte count"
              # "Read byte count"
              n211 = Format Into String(format string=":CALC:PN:TRAC1:DATA:U%s?;", w795) -> (resulting string=w809:string)  [unwired: 2 in, 1 out]
              n212 = VISA Write(VISA resource name=w794, write buffer=w809, error in (no error)=w793) -> (VISA resource name out=w800:refnum<visa-resource-name>, error out=w799:errorcluster)  [unwired: 1 out]
              n213 = VISA Read(VISA resource name=w800, byte count=u32 2, error in (no error)=w799) -> (VISA resource name out=w805:refnum<visa-resource-name>, read buffer=w801:string, error out=w806:errorcluster)  [unwired: 1 out]
              n214 = Scan From String(format string="#%1d", input string=w801) -> (output 1=w804:i32)  [unwired: 3 in, 3 out]
              n215 = VISA Read(VISA resource name=w805, byte count=w804, error in (no error)=w806) -> (VISA resource name out=w798:refnum<visa-resource-name>, read buffer=w803:string, error out=w797:errorcluster)  [unwired: 1 out]
              n216 = Scan From String(format string="%d", input string=w803) -> (output 1=w796:i32)  [unwired: 3 in, 3 out]
              n217 = VISA Read(VISA resource name=w798, byte count=w796, error in (no error)=w797) -> (VISA resource name out=w792:refnum<visa-resource-name>, read buffer=w790:string, error out=w791:errorcluster)  [unwired: 1 out]
            }
            frame "Power" {
              # "Read num digits in byte count"
              # "Read byte count"
              n218 = Format Into String(format string=":CALC:PN:TRAC1:DATA:P%s?;", w816) -> (resulting string=w830:string)  [unwired: 2 in, 1 out]
              n219 = VISA Write(VISA resource name=w815, write buffer=w830, error in (no error)=w814) -> (VISA resource name out=w821:refnum<visa-resource-name>, error out=w820:errorcluster)  [unwired: 1 out]
              n220 = VISA Read(VISA resource name=w821, byte count=u32 2, error in (no error)=w820) -> (VISA resource name out=w826:refnum<visa-resource-name>, read buffer=w822:string, error out=w827:errorcluster)  [unwired: 1 out]
              n221 = Scan From String(format string="#%1d", input string=w822) -> (output 1=w825:i32)  [unwired: 3 in, 3 out]
              n222 = VISA Read(VISA resource name=w826, byte count=w825, error in (no error)=w827) -> (VISA resource name out=w819:refnum<visa-resource-name>, read buffer=w824:string, error out=w818:errorcluster)  [unwired: 1 out]
              n223 = Scan From String(format string="%d", input string=w824) -> (output 1=w817:i32)  [unwired: 3 in, 3 out]
              n224 = VISA Read(VISA resource name=w819, byte count=w817, error in (no error)=w818) -> (VISA resource name out=w813:refnum<visa-resource-name>, read buffer=w812:string, error out=w811:errorcluster)  [unwired: 1 out]
            }
            frame "Spurious" {
              # "Read num digits in byte count"
              # "Read byte count"
              n225 = Format Into String(format string=":CALC:PN:TRAC1:DATA:S%s?;", w837) -> (resulting string=w851:string)  [unwired: 2 in, 1 out]
              n226 = VISA Write(VISA resource name=w836, write buffer=w851, error in (no error)=w835) -> (VISA resource name out=w842:refnum<visa-resource-name>, error out=w841:errorcluster)  [unwired: 1 out]
              n227 = VISA Read(VISA resource name=w842, byte count=u32 2, error in (no error)=w841) -> (VISA resource name out=w847:refnum<visa-resource-name>, read buffer=w843:string, error out=w848:errorcluster)  [unwired: 1 out]
              n228 = Scan From String(format string="#%1d", input string=w843) -> (output 1=w846:i32)  [unwired: 3 in, 3 out]
              n229 = VISA Read(VISA resource name=w847, byte count=w846, error in (no error)=w848) -> (VISA resource name out=w840:refnum<visa-resource-name>, read buffer=w845:string, error out=w839:errorcluster)  [unwired: 1 out]
              n230 = Scan From String(format string="%d", input string=w845) -> (output 1=w838:i32)  [unwired: 3 in, 3 out]
              n231 = VISA Read(VISA resource name=w840, byte count=w838, error in (no error)=w839) -> (VISA resource name out=w834:refnum<visa-resource-name>, read buffer=w832:string, error out=w833:errorcluster)  [unwired: 1 out]
            }
          }
        }
        frame 2..8 {
          # "Trace 2-8"
        }
      }
    }
    frame 7 {
      # "User"
      n232 = case shown="1, Default" w861 {
        tunnel: w862 -> [w869 w924 w979 w1034 w1089 w1144 w1199 w1254]
        tunnel: w863 -> [w870 w925 w980 w1035 w1090 w1145 w1200 w1255]
        tunnel: w860 -> [w868 w923 w978 w1033 w1088 w1143 w1198 w1253]
        tunnel: w859 -> [w867 w922 w977 w1032 w1087 w1142 w1197 w1252]
        tunnel: [w866 w921 w976 w1031 w1086 w1141 w1196 w1251] -> w858
        tunnel: [w865 w920 w975 w1030 w1085 w1140 w1195 w1250] -> w856
        tunnel: [w864 w919 w974 w1029 w1084 w1139 w1194 w1249] -> w857
        frame 1, Default {
          # "Trace 1"
          n233 = case shown="\"Formatted\", Default" w870 {
            tunnel: w869 -> [w890 w897 _ _]
            tunnel: w868 -> [w889 w896 w915 w918]
            tunnel: w867 -> [w888 w895 w914 w917]
            tunnel: [w886 w894 w915 w918] -> w866
            tunnel: [w885 w893 w914 w917] -> w865
            tunnel: [w884 w892 "" ""] -> w864
            frame "Formatted", Default {
              # "Read num digits in byte count"
              # "Read byte count"
              n234 = Format Into String(format string=":CALC:USER:TRAC1:DATA:F%s?;", w890) -> (resulting string=w887:string)  [unwired: 2 in, 1 out]
              n235 = VISA Write(VISA resource name=w889, write buffer=w887, error in (no error)=w888) -> (VISA resource name out=w875:refnum<visa-resource-name>, error out=w874:errorcluster)  [unwired: 1 out]
              n236 = VISA Read(VISA resource name=w875, byte count=u32 2, error in (no error)=w874) -> (VISA resource name out=w880:refnum<visa-resource-name>, read buffer=w876:string, error out=w881:errorcluster)  [unwired: 1 out]
              n237 = Scan From String(format string="#%1d", input string=w876) -> (output 1=w879:i32)  [unwired: 3 in, 3 out]
              n238 = VISA Read(VISA resource name=w880, byte count=w879, error in (no error)=w881) -> (VISA resource name out=w873:refnum<visa-resource-name>, read buffer=w878:string, error out=w872:errorcluster)  [unwired: 1 out]
              n239 = Scan From String(format string="%d", input string=w878) -> (output 1=w871:i32)  [unwired: 3 in, 3 out]
              n240 = VISA Read(VISA resource name=w873, byte count=w871, error in (no error)=w872) -> (VISA resource name out=w886:refnum<visa-resource-name>, read buffer=w884:string, error out=w885:errorcluster)  [unwired: 1 out]
            }
            frame "Unformatted" {
              # "Read num digits in byte count"
              # "Read byte count"
              n241 = Format Into String(format string=":CALC:USER:TRAC1:DATA:U%s?;", w897) -> (resulting string=w911:string)  [unwired: 2 in, 1 out]
              n242 = VISA Write(VISA resource name=w896, write buffer=w911, error in (no error)=w895) -> (VISA resource name out=w902:refnum<visa-resource-name>, error out=w901:errorcluster)  [unwired: 1 out]
              n243 = VISA Read(VISA resource name=w902, byte count=u32 2, error in (no error)=w901) -> (VISA resource name out=w907:refnum<visa-resource-name>, read buffer=w903:string, error out=w908:errorcluster)  [unwired: 1 out]
              n244 = Scan From String(format string="#%1d", input string=w903) -> (output 1=w906:i32)  [unwired: 3 in, 3 out]
              n245 = VISA Read(VISA resource name=w907, byte count=w906, error in (no error)=w908) -> (VISA resource name out=w900:refnum<visa-resource-name>, read buffer=w905:string, error out=w899:errorcluster)  [unwired: 1 out]
              n246 = Scan From String(format string="%d", input string=w905) -> (output 1=w898:i32)  [unwired: 3 in, 3 out]
              n247 = VISA Read(VISA resource name=w900, byte count=w898, error in (no error)=w899) -> (VISA resource name out=w894:refnum<visa-resource-name>, read buffer=w892:string, error out=w893:errorcluster)  [unwired: 1 out]
            }
            frame "Power" {
            }
            frame "Spurious" {
            }
          }
        }
        frame 2 {
          # "Trace 2"
          n248 = case shown="\"Formatted\", Default" w925 {
            tunnel: w924 -> [w945 w952 _ _]
            tunnel: w923 -> [w944 w951 w970 w973]
            tunnel: w922 -> [w943 w950 w969 w972]
            tunnel: [w941 w949 w970 w973] -> w921
            tunnel: [w940 w948 w969 w972] -> w920
            tunnel: [w939 w947 "" ""] -> w919
            frame "Formatted", Default {
              # "Read num digits in byte count"
              # "Read byte count"
              n249 = Format Into String(format string=":CALC:USER:TRAC2:DATA:F%s?;", w945) -> (resulting string=w942:string)  [unwired: 2 in, 1 out]
              n250 = VISA Write(VISA resource name=w944, write buffer=w942, error in (no error)=w943) -> (VISA resource name out=w930:refnum<visa-resource-name>, error out=w929:errorcluster)  [unwired: 1 out]
              n251 = VISA Read(VISA resource name=w930, byte count=u32 2, error in (no error)=w929) -> (VISA resource name out=w935:refnum<visa-resource-name>, read buffer=w931:string, error out=w936:errorcluster)  [unwired: 1 out]
              n252 = Scan From String(format string="#%1d", input string=w931) -> (output 1=w934:i32)  [unwired: 3 in, 3 out]
              n253 = VISA Read(VISA resource name=w935, byte count=w934, error in (no error)=w936) -> (VISA resource name out=w928:refnum<visa-resource-name>, read buffer=w933:string, error out=w927:errorcluster)  [unwired: 1 out]
              n254 = Scan From String(format string="%d", input string=w933) -> (output 1=w926:i32)  [unwired: 3 in, 3 out]
              n255 = VISA Read(VISA resource name=w928, byte count=w926, error in (no error)=w927) -> (VISA resource name out=w941:refnum<visa-resource-name>, read buffer=w939:string, error out=w940:errorcluster)  [unwired: 1 out]
            }
            frame "Unformatted" {
              # "Read num digits in byte count"
              # "Read byte count"
              n256 = Format Into String(format string=":CALC:USER:TRAC2:DATA:U%s?;", w952) -> (resulting string=w966:string)  [unwired: 2 in, 1 out]
              n257 = VISA Write(VISA resource name=w951, write buffer=w966, error in (no error)=w950) -> (VISA resource name out=w957:refnum<visa-resource-name>, error out=w956:errorcluster)  [unwired: 1 out]
              n258 = VISA Read(VISA resource name=w957, byte count=u32 2, error in (no error)=w956) -> (VISA resource name out=w962:refnum<visa-resource-name>, read buffer=w958:string, error out=w963:errorcluster)  [unwired: 1 out]
              n259 = Scan From String(format string="#%1d", input string=w958) -> (output 1=w961:i32)  [unwired: 3 in, 3 out]
              n260 = VISA Read(VISA resource name=w962, byte count=w961, error in (no error)=w963) -> (VISA resource name out=w955:refnum<visa-resource-name>, read buffer=w960:string, error out=w954:errorcluster)  [unwired: 1 out]
              n261 = Scan From String(format string="%d", input string=w960) -> (output 1=w953:i32)  [unwired: 3 in, 3 out]
              n262 = VISA Read(VISA resource name=w955, byte count=w953, error in (no error)=w954) -> (VISA resource name out=w949:refnum<visa-resource-name>, read buffer=w947:string, error out=w948:errorcluster)  [unwired: 1 out]
            }
            frame "Power" {
            }
            frame "Spurious" {
            }
          }
        }
        frame 3 {
          # "Trace 3"
          n263 = case shown="\"Formatted\", Default" w980 {
            tunnel: w979 -> [w1000 w1007 _ _]
            tunnel: w978 -> [w999 w1006 w1025 w1028]
            tunnel: w977 -> [w998 w1005 w1024 w1027]
            tunnel: [w996 w1004 w1025 w1028] -> w976
            tunnel: [w995 w1003 w1024 w1027] -> w975
            tunnel: [w994 w1002 "" ""] -> w974
            frame "Formatted", Default {
              # "Read num digits in byte count"
              # "Read byte count"
              n264 = Format Into String(format string=":CALC:USER:TRAC3:DATA:F%s?;", w1000) -> (resulting string=w997:string)  [unwired: 2 in, 1 out]
              n265 = VISA Write(VISA resource name=w999, write buffer=w997, error in (no error)=w998) -> (VISA resource name out=w985:refnum<visa-resource-name>, error out=w984:errorcluster)  [unwired: 1 out]
              n266 = VISA Read(VISA resource name=w985, byte count=u32 2, error in (no error)=w984) -> (VISA resource name out=w990:refnum<visa-resource-name>, read buffer=w986:string, error out=w991:errorcluster)  [unwired: 1 out]
              n267 = Scan From String(format string="#%1d", input string=w986) -> (output 1=w989:i32)  [unwired: 3 in, 3 out]
              n268 = VISA Read(VISA resource name=w990, byte count=w989, error in (no error)=w991) -> (VISA resource name out=w983:refnum<visa-resource-name>, read buffer=w988:string, error out=w982:errorcluster)  [unwired: 1 out]
              n269 = Scan From String(format string="%d", input string=w988) -> (output 1=w981:i32)  [unwired: 3 in, 3 out]
              n270 = VISA Read(VISA resource name=w983, byte count=w981, error in (no error)=w982) -> (VISA resource name out=w996:refnum<visa-resource-name>, read buffer=w994:string, error out=w995:errorcluster)  [unwired: 1 out]
            }
            frame "Unformatted" {
              # "Read num digits in byte count"
              # "Read byte count"
              n271 = Format Into String(format string=":CALC:USER:TRAC3:DATA:U%s?;", w1007) -> (resulting string=w1021:string)  [unwired: 2 in, 1 out]
              n272 = VISA Write(VISA resource name=w1006, write buffer=w1021, error in (no error)=w1005) -> (VISA resource name out=w1012:refnum<visa-resource-name>, error out=w1011:errorcluster)  [unwired: 1 out]
              n273 = VISA Read(VISA resource name=w1012, byte count=u32 2, error in (no error)=w1011) -> (VISA resource name out=w1017:refnum<visa-resource-name>, read buffer=w1013:string, error out=w1018:errorcluster)  [unwired: 1 out]
              n274 = Scan From String(format string="#%1d", input string=w1013) -> (output 1=w1016:i32)  [unwired: 3 in, 3 out]
              n275 = VISA Read(VISA resource name=w1017, byte count=w1016, error in (no error)=w1018) -> (VISA resource name out=w1010:refnum<visa-resource-name>, read buffer=w1015:string, error out=w1009:errorcluster)  [unwired: 1 out]
              n276 = Scan From String(format string="%d", input string=w1015) -> (output 1=w1008:i32)  [unwired: 3 in, 3 out]
              n277 = VISA Read(VISA resource name=w1010, byte count=w1008, error in (no error)=w1009) -> (VISA resource name out=w1004:refnum<visa-resource-name>, read buffer=w1002:string, error out=w1003:errorcluster)  [unwired: 1 out]
            }
            frame "Power" {
            }
            frame "Spurious" {
            }
          }
        }
        frame 4 {
          # "Trace 4"
          n278 = case shown="\"Formatted\", Default" w1035 {
            tunnel: w1034 -> [w1055 w1062 _ _]
            tunnel: w1033 -> [w1054 w1061 w1080 w1083]
            tunnel: w1032 -> [w1053 w1060 w1079 w1082]
            tunnel: [w1051 w1059 w1080 w1083] -> w1031
            tunnel: [w1050 w1058 w1079 w1082] -> w1030
            tunnel: [w1049 w1057 "" ""] -> w1029
            frame "Formatted", Default {
              # "Read num digits in byte count"
              # "Read byte count"
              n279 = Format Into String(format string=":CALC:USER:TRAC4:DATA:F%s?;", w1055) -> (resulting string=w1052:string)  [unwired: 2 in, 1 out]
              n280 = VISA Write(VISA resource name=w1054, write buffer=w1052, error in (no error)=w1053) -> (VISA resource name out=w1040:refnum<visa-resource-name>, error out=w1039:errorcluster)  [unwired: 1 out]
              n281 = VISA Read(VISA resource name=w1040, byte count=u32 2, error in (no error)=w1039) -> (VISA resource name out=w1045:refnum<visa-resource-name>, read buffer=w1041:string, error out=w1046:errorcluster)  [unwired: 1 out]
              n282 = Scan From String(format string="#%1d", input string=w1041) -> (output 1=w1044:i32)  [unwired: 3 in, 3 out]
              n283 = VISA Read(VISA resource name=w1045, byte count=w1044, error in (no error)=w1046) -> (VISA resource name out=w1038:refnum<visa-resource-name>, read buffer=w1043:string, error out=w1037:errorcluster)  [unwired: 1 out]
              n284 = Scan From String(format string="%d", input string=w1043) -> (output 1=w1036:i32)  [unwired: 3 in, 3 out]
              n285 = VISA Read(VISA resource name=w1038, byte count=w1036, error in (no error)=w1037) -> (VISA resource name out=w1051:refnum<visa-resource-name>, read buffer=w1049:string, error out=w1050:errorcluster)  [unwired: 1 out]
            }
            frame "Unformatted" {
              # "Read num digits in byte count"
              # "Read byte count"
              n286 = Format Into String(format string=":CALC:USER:TRAC4:DATA:U%s?;", w1062) -> (resulting string=w1076:string)  [unwired: 2 in, 1 out]
              n287 = VISA Write(VISA resource name=w1061, write buffer=w1076, error in (no error)=w1060) -> (VISA resource name out=w1067:refnum<visa-resource-name>, error out=w1066:errorcluster)  [unwired: 1 out]
              n288 = VISA Read(VISA resource name=w1067, byte count=u32 2, error in (no error)=w1066) -> (VISA resource name out=w1072:refnum<visa-resource-name>, read buffer=w1068:string, error out=w1073:errorcluster)  [unwired: 1 out]
              n289 = Scan From String(format string="#%1d", input string=w1068) -> (output 1=w1071:i32)  [unwired: 3 in, 3 out]
              n290 = VISA Read(VISA resource name=w1072, byte count=w1071, error in (no error)=w1073) -> (VISA resource name out=w1065:refnum<visa-resource-name>, read buffer=w1070:string, error out=w1064:errorcluster)  [unwired: 1 out]
              n291 = Scan From String(format string="%d", input string=w1070) -> (output 1=w1063:i32)  [unwired: 3 in, 3 out]
              n292 = VISA Read(VISA resource name=w1065, byte count=w1063, error in (no error)=w1064) -> (VISA resource name out=w1059:refnum<visa-resource-name>, read buffer=w1057:string, error out=w1058:errorcluster)  [unwired: 1 out]
            }
            frame "Power" {
            }
            frame "Spurious" {
            }
          }
        }
        frame 5 {
          # "Trace 5"
          n293 = case shown="\"Formatted\", Default" w1090 {
            tunnel: w1089 -> [w1110 w1117 _ _]
            tunnel: w1088 -> [w1109 w1116 w1135 w1138]
            tunnel: w1087 -> [w1108 w1115 w1134 w1137]
            tunnel: [w1106 w1114 w1135 w1138] -> w1086
            tunnel: [w1105 w1113 w1134 w1137] -> w1085
            tunnel: [w1104 w1112 "" ""] -> w1084
            frame "Formatted", Default {
              # "Read num digits in byte count"
              # "Read byte count"
              n294 = Format Into String(format string=":CALC:USER:TRAC5:DATA:F%s?;", w1110) -> (resulting string=w1107:string)  [unwired: 2 in, 1 out]
              n295 = VISA Write(VISA resource name=w1109, write buffer=w1107, error in (no error)=w1108) -> (VISA resource name out=w1095:refnum<visa-resource-name>, error out=w1094:errorcluster)  [unwired: 1 out]
              n296 = VISA Read(VISA resource name=w1095, byte count=u32 2, error in (no error)=w1094) -> (VISA resource name out=w1100:refnum<visa-resource-name>, read buffer=w1096:string, error out=w1101:errorcluster)  [unwired: 1 out]
              n297 = Scan From String(format string="#%1d", input string=w1096) -> (output 1=w1099:i32)  [unwired: 3 in, 3 out]
              n298 = VISA Read(VISA resource name=w1100, byte count=w1099, error in (no error)=w1101) -> (VISA resource name out=w1093:refnum<visa-resource-name>, read buffer=w1098:string, error out=w1092:errorcluster)  [unwired: 1 out]
              n299 = Scan From String(format string="%d", input string=w1098) -> (output 1=w1091:i32)  [unwired: 3 in, 3 out]
              n300 = VISA Read(VISA resource name=w1093, byte count=w1091, error in (no error)=w1092) -> (VISA resource name out=w1106:refnum<visa-resource-name>, read buffer=w1104:string, error out=w1105:errorcluster)  [unwired: 1 out]
            }
            frame "Unformatted" {
              # "Read num digits in byte count"
              # "Read byte count"
              n301 = Format Into String(format string=":CALC:USER:TRAC5:DATA:U%s?;", w1117) -> (resulting string=w1131:string)  [unwired: 2 in, 1 out]
              n302 = VISA Write(VISA resource name=w1116, write buffer=w1131, error in (no error)=w1115) -> (VISA resource name out=w1122:refnum<visa-resource-name>, error out=w1121:errorcluster)  [unwired: 1 out]
              n303 = VISA Read(VISA resource name=w1122, byte count=u32 2, error in (no error)=w1121) -> (VISA resource name out=w1127:refnum<visa-resource-name>, read buffer=w1123:string, error out=w1128:errorcluster)  [unwired: 1 out]
              n304 = Scan From String(format string="#%1d", input string=w1123) -> (output 1=w1126:i32)  [unwired: 3 in, 3 out]
              n305 = VISA Read(VISA resource name=w1127, byte count=w1126, error in (no error)=w1128) -> (VISA resource name out=w1120:refnum<visa-resource-name>, read buffer=w1125:string, error out=w1119:errorcluster)  [unwired: 1 out]
              n306 = Scan From String(format string="%d", input string=w1125) -> (output 1=w1118:i32)  [unwired: 3 in, 3 out]
              n307 = VISA Read(VISA resource name=w1120, byte count=w1118, error in (no error)=w1119) -> (VISA resource name out=w1114:refnum<visa-resource-name>, read buffer=w1112:string, error out=w1113:errorcluster)  [unwired: 1 out]
            }
            frame "Power" {
            }
            frame "Spurious" {
            }
          }
        }
        frame 6 {
          # "Trace 6"
          n308 = case shown="\"Formatted\", Default" w1145 {
            tunnel: w1144 -> [w1165 w1172 _ _]
            tunnel: w1143 -> [w1164 w1171 w1190 w1193]
            tunnel: w1142 -> [w1163 w1170 w1189 w1192]
            tunnel: [w1161 w1169 w1190 w1193] -> w1141
            tunnel: [w1160 w1168 w1189 w1192] -> w1140
            tunnel: [w1159 w1167 "" ""] -> w1139
            frame "Formatted", Default {
              # "Read num digits in byte count"
              # "Read byte count"
              n309 = Format Into String(format string=":CALC:USER:TRAC6:DATA:F%s?;", w1165) -> (resulting string=w1162:string)  [unwired: 2 in, 1 out]
              n310 = VISA Write(VISA resource name=w1164, write buffer=w1162, error in (no error)=w1163) -> (VISA resource name out=w1150:refnum<visa-resource-name>, error out=w1149:errorcluster)  [unwired: 1 out]
              n311 = VISA Read(VISA resource name=w1150, byte count=u32 2, error in (no error)=w1149) -> (VISA resource name out=w1155:refnum<visa-resource-name>, read buffer=w1151:string, error out=w1156:errorcluster)  [unwired: 1 out]
              n312 = Scan From String(format string="#%1d", input string=w1151) -> (output 1=w1154:i32)  [unwired: 3 in, 3 out]
              n313 = VISA Read(VISA resource name=w1155, byte count=w1154, error in (no error)=w1156) -> (VISA resource name out=w1148:refnum<visa-resource-name>, read buffer=w1153:string, error out=w1147:errorcluster)  [unwired: 1 out]
              n314 = Scan From String(format string="%d", input string=w1153) -> (output 1=w1146:i32)  [unwired: 3 in, 3 out]
              n315 = VISA Read(VISA resource name=w1148, byte count=w1146, error in (no error)=w1147) -> (VISA resource name out=w1161:refnum<visa-resource-name>, read buffer=w1159:string, error out=w1160:errorcluster)  [unwired: 1 out]
            }
            frame "Unformatted" {
              # "Read num digits in byte count"
              # "Read byte count"
              n316 = Format Into String(format string=":CALC:USER:TRAC6:DATA:U%s?;", w1172) -> (resulting string=w1186:string)  [unwired: 2 in, 1 out]
              n317 = VISA Write(VISA resource name=w1171, write buffer=w1186, error in (no error)=w1170) -> (VISA resource name out=w1177:refnum<visa-resource-name>, error out=w1176:errorcluster)  [unwired: 1 out]
              n318 = VISA Read(VISA resource name=w1177, byte count=u32 2, error in (no error)=w1176) -> (VISA resource name out=w1182:refnum<visa-resource-name>, read buffer=w1178:string, error out=w1183:errorcluster)  [unwired: 1 out]
              n319 = Scan From String(format string="#%1d", input string=w1178) -> (output 1=w1181:i32)  [unwired: 3 in, 3 out]
              n320 = VISA Read(VISA resource name=w1182, byte count=w1181, error in (no error)=w1183) -> (VISA resource name out=w1175:refnum<visa-resource-name>, read buffer=w1180:string, error out=w1174:errorcluster)  [unwired: 1 out]
              n321 = Scan From String(format string="%d", input string=w1180) -> (output 1=w1173:i32)  [unwired: 3 in, 3 out]
              n322 = VISA Read(VISA resource name=w1175, byte count=w1173, error in (no error)=w1174) -> (VISA resource name out=w1169:refnum<visa-resource-name>, read buffer=w1167:string, error out=w1168:errorcluster)  [unwired: 1 out]
            }
            frame "Power" {
            }
            frame "Spurious" {
            }
          }
        }
        frame 7 {
          # "Trace 7"
          n323 = case shown="\"Formatted\", Default" w1200 {
            tunnel: w1199 -> [w1220 w1227 _ _]
            tunnel: w1198 -> [w1219 w1226 w1245 w1248]
            tunnel: w1197 -> [w1218 w1225 w1244 w1247]
            tunnel: [w1216 w1224 w1245 w1248] -> w1196
            tunnel: [w1215 w1223 w1244 w1247] -> w1195
            tunnel: [w1214 w1222 "" ""] -> w1194
            frame "Formatted", Default {
              # "Read num digits in byte count"
              # "Read byte count"
              n324 = Format Into String(format string=":CALC:USER:TRAC7:DATA:F%s?;", w1220) -> (resulting string=w1217:string)  [unwired: 2 in, 1 out]
              n325 = VISA Write(VISA resource name=w1219, write buffer=w1217, error in (no error)=w1218) -> (VISA resource name out=w1205:refnum<visa-resource-name>, error out=w1204:errorcluster)  [unwired: 1 out]
              n326 = VISA Read(VISA resource name=w1205, byte count=u32 2, error in (no error)=w1204) -> (VISA resource name out=w1210:refnum<visa-resource-name>, read buffer=w1206:string, error out=w1211:errorcluster)  [unwired: 1 out]
              n327 = Scan From String(format string="#%1d", input string=w1206) -> (output 1=w1209:i32)  [unwired: 3 in, 3 out]
              n328 = VISA Read(VISA resource name=w1210, byte count=w1209, error in (no error)=w1211) -> (VISA resource name out=w1203:refnum<visa-resource-name>, read buffer=w1208:string, error out=w1202:errorcluster)  [unwired: 1 out]
              n329 = Scan From String(format string="%d", input string=w1208) -> (output 1=w1201:i32)  [unwired: 3 in, 3 out]
              n330 = VISA Read(VISA resource name=w1203, byte count=w1201, error in (no error)=w1202) -> (VISA resource name out=w1216:refnum<visa-resource-name>, read buffer=w1214:string, error out=w1215:errorcluster)  [unwired: 1 out]
            }
            frame "Unformatted" {
              # "Read num digits in byte count"
              # "Read byte count"
              n331 = Format Into String(format string=":CALC:USER:TRAC7:DATA:U%s?;", w1227) -> (resulting string=w1241:string)  [unwired: 2 in, 1 out]
              n332 = VISA Write(VISA resource name=w1226, write buffer=w1241, error in (no error)=w1225) -> (VISA resource name out=w1232:refnum<visa-resource-name>, error out=w1231:errorcluster)  [unwired: 1 out]
              n333 = VISA Read(VISA resource name=w1232, byte count=u32 2, error in (no error)=w1231) -> (VISA resource name out=w1237:refnum<visa-resource-name>, read buffer=w1233:string, error out=w1238:errorcluster)  [unwired: 1 out]
              n334 = Scan From String(format string="#%1d", input string=w1233) -> (output 1=w1236:i32)  [unwired: 3 in, 3 out]
              n335 = VISA Read(VISA resource name=w1237, byte count=w1236, error in (no error)=w1238) -> (VISA resource name out=w1230:refnum<visa-resource-name>, read buffer=w1235:string, error out=w1229:errorcluster)  [unwired: 1 out]
              n336 = Scan From String(format string="%d", input string=w1235) -> (output 1=w1228:i32)  [unwired: 3 in, 3 out]
              n337 = VISA Read(VISA resource name=w1230, byte count=w1228, error in (no error)=w1229) -> (VISA resource name out=w1224:refnum<visa-resource-name>, read buffer=w1222:string, error out=w1223:errorcluster)  [unwired: 1 out]
            }
            frame "Power" {
            }
            frame "Spurious" {
            }
          }
        }
        frame 8 {
          # "Trace 8"
          n338 = case shown="\"Formatted\", Default" w1255 {
            tunnel: w1254 -> [w1275 w1282 _ _]
            tunnel: w1253 -> [w1274 w1281 w1300 w1303]
            tunnel: w1252 -> [w1273 w1280 w1299 w1302]
            tunnel: [w1271 w1279 w1300 w1303] -> w1251
            tunnel: [w1270 w1278 w1299 w1302] -> w1250
            tunnel: [w1269 w1277 "" ""] -> w1249
            frame "Formatted", Default {
              # "Read num digits in byte count"
              # "Read byte count"
              n339 = Format Into String(format string=":CALC:USER:TRAC8:DATA:F%s?;", w1275) -> (resulting string=w1272:string)  [unwired: 2 in, 1 out]
              n340 = VISA Write(VISA resource name=w1274, write buffer=w1272, error in (no error)=w1273) -> (VISA resource name out=w1260:refnum<visa-resource-name>, error out=w1259:errorcluster)  [unwired: 1 out]
              n341 = VISA Read(VISA resource name=w1260, byte count=u32 2, error in (no error)=w1259) -> (VISA resource name out=w1265:refnum<visa-resource-name>, read buffer=w1261:string, error out=w1266:errorcluster)  [unwired: 1 out]
              n342 = Scan From String(format string="#%1d", input string=w1261) -> (output 1=w1264:i32)  [unwired: 3 in, 3 out]
              n343 = VISA Read(VISA resource name=w1265, byte count=w1264, error in (no error)=w1266) -> (VISA resource name out=w1258:refnum<visa-resource-name>, read buffer=w1263:string, error out=w1257:errorcluster)  [unwired: 1 out]
              n344 = Scan From String(format string="%d", input string=w1263) -> (output 1=w1256:i32)  [unwired: 3 in, 3 out]
              n345 = VISA Read(VISA resource name=w1258, byte count=w1256, error in (no error)=w1257) -> (VISA resource name out=w1271:refnum<visa-resource-name>, read buffer=w1269:string, error out=w1270:errorcluster)  [unwired: 1 out]
            }
            frame "Unformatted" {
              # "Read num digits in byte count"
              # "Read byte count"
              n346 = Format Into String(format string=":CALC:USER:TRAC8:DATA:U%s?;", w1282) -> (resulting string=w1296:string)  [unwired: 2 in, 1 out]
              n347 = VISA Write(VISA resource name=w1281, write buffer=w1296, error in (no error)=w1280) -> (VISA resource name out=w1287:refnum<visa-resource-name>, error out=w1286:errorcluster)  [unwired: 1 out]
              n348 = VISA Read(VISA resource name=w1287, byte count=u32 2, error in (no error)=w1286) -> (VISA resource name out=w1292:refnum<visa-resource-name>, read buffer=w1288:string, error out=w1293:errorcluster)  [unwired: 1 out]
              n349 = Scan From String(format string="#%1d", input string=w1288) -> (output 1=w1291:i32)  [unwired: 3 in, 3 out]
              n350 = VISA Read(VISA resource name=w1292, byte count=w1291, error in (no error)=w1293) -> (VISA resource name out=w1285:refnum<visa-resource-name>, read buffer=w1290:string, error out=w1284:errorcluster)  [unwired: 1 out]
              n351 = Scan From String(format string="%d", input string=w1290) -> (output 1=w1283:i32)  [unwired: 3 in, 3 out]
              n352 = VISA Read(VISA resource name=w1285, byte count=w1283, error in (no error)=w1284) -> (VISA resource name out=w1279:refnum<visa-resource-name>, read buffer=w1277:string, error out=w1278:errorcluster)  [unwired: 1 out]
            }
            frame "Power" {
            }
            frame "Spurious" {
            }
          }
        }
      }
    }
  }
  n353 = VISA Clear(VISA resource name=w13, error in (no error)=w12) -> (VISA resource name out=w11:refnum<visa-resource-name>, error out=w10:errorcluster)
  n354 = Build Array(sgl 0.0) -> (w3:sgl[])
  n355 = Type Cast(type=w3, x=w2) -> (*(type *) &x=→"Measurements":sgl[])
  n356 = call "Error Query.vi"("error in (no error)"=w10, "VISA resource name"=w11) -> ("error out"=→"error out":errorcluster, "VISA resource name out"=→"VISA resource name out":refnum<visa-resource-name>)  [unwired: 6 in, 2 out]
